vi "子界面-图像预处理.vi"(11 "原图":T1(plugin-control)) -> (3 "处理后":T1(plugin-control))   [LabVIEW 2018]
uses:
  <vilib>/vision/NI_Vision_Development_Module.lvlib
panel:
  in  "返回":bool
  in  "确认":bool
  in  "结构元素":i32[][](array[numeric])=[[1, 1, 1], [1, 1, 1], [1, 1, 1]]
  in  "处理模式":T2(ring)
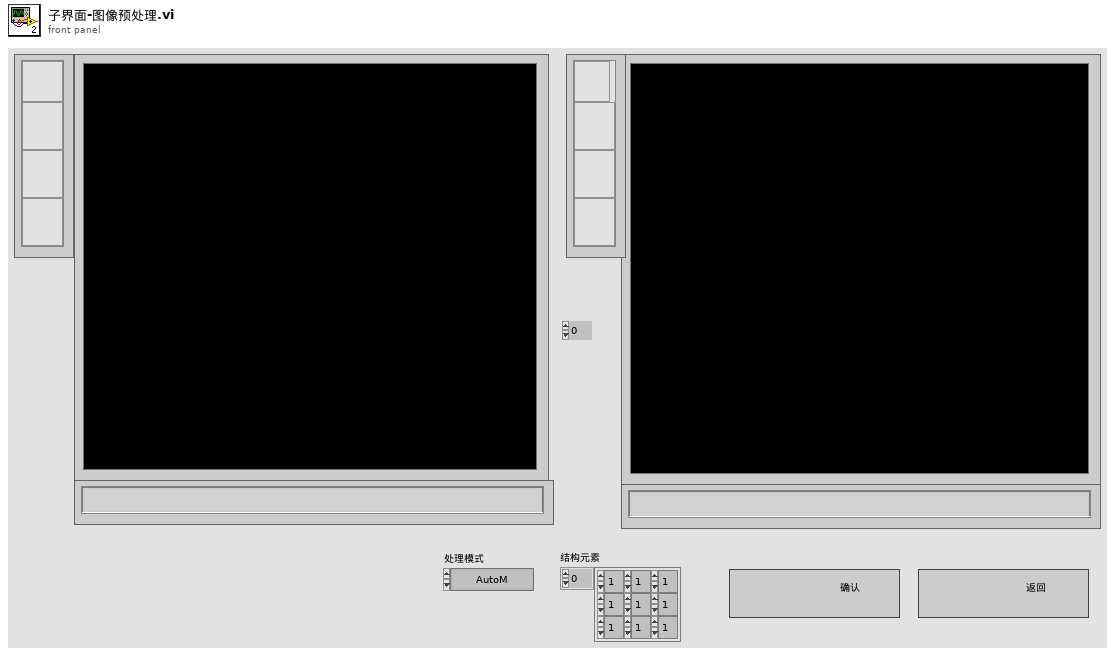
[diagram p1: front panel]
types:
  T1 = typedef "IMAQ Image.ctl" = refnum<image>
  T2 = enum32{"AutoM", "Close", "Dilate", "Erode", "Gradient", "Gradient in", "Gradient out", "HitMiss", "Open", "PClose", "POpen", "Thick", "Thin"}
  T3 = typedef "Image Type" = u32
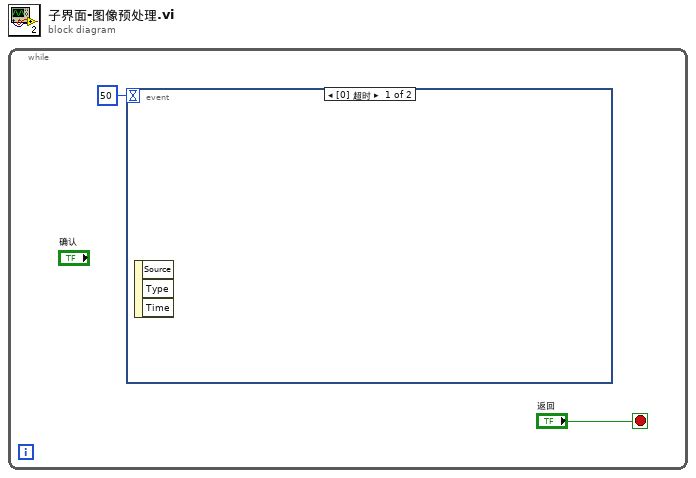
[diagram p0: block diagram]
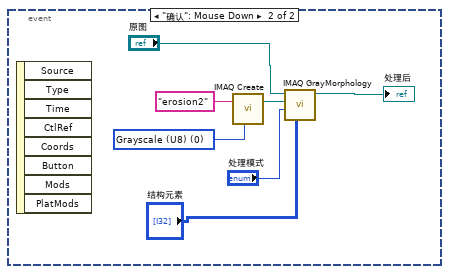
[diagram p2: hidden frame]
diagram:
  n1 = while {
    stop <- "返回" stop-if-true
    n2 = event shown="[0] 超时" {
      selector: _ -> [_ _]
      dyn-events: _ -> [_ _]
      timeout: 50 -> [_ _]
      event Timeout {
        n3 = event-data() -> ()  [unwired: 1 in, 3 out]
      }
      event "确认": Mouse Down {
        w4 = T3 0 items=["Grayscale (U8)", "Grayscale (I16)", "Grayscale (SGL)", "Complex (CSG)", "RGB (U32)", "HSL (U32)", "RGB (U64)", "Grayscale (U16)"] ("Image Type")
        n4 = event-data() -> ()  [unwired: 1 in, 8 out]
        n5 = call "IMAQ Create"("Image Name"="erosion2", "Image Type"=w4) -> ("New Image"=w8:T1)  [unwired: 3 in, 1 out]
        n6 = call "IMAQ GrayMorphology"("Structuring Element"="结构元素", "Operation"="处理模式", "Image Dst"=w8, "Image Src"="原图") -> ("Image Dst Out"=→"处理后":T1)  [unwired: 6 in, 1 out]
      }
    }
  }
